vi "Get or Add Borders.vi"(8 "error in":errorcluster, 11 "SpreadsheetDoc in":refnum<k24>) -> (0 "error out":errorcluster, 2 "Borders":refnum<k24>, 3 "SpreadsheetDoc out":refnum<k24>)   [LabVIEW 2019, in "Open Xml.lvlib"]
uses:
  Open Xml.lvlib
  D:/git/Open-Xml-LabVIEW/Source/DocumentFormat.OpenXml.dll
  DocumentFormat.OpenXml.dll
  D:/git/Open-Xml-LabVIEW/Source/DocumentFormat.OpenXml.Framework.dll
  DocumentFormat.OpenXml.Framework.dll
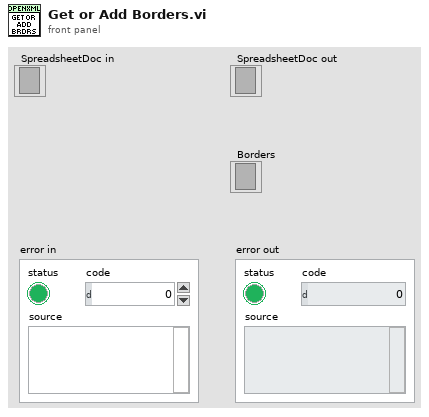
[diagram p1: front panel]
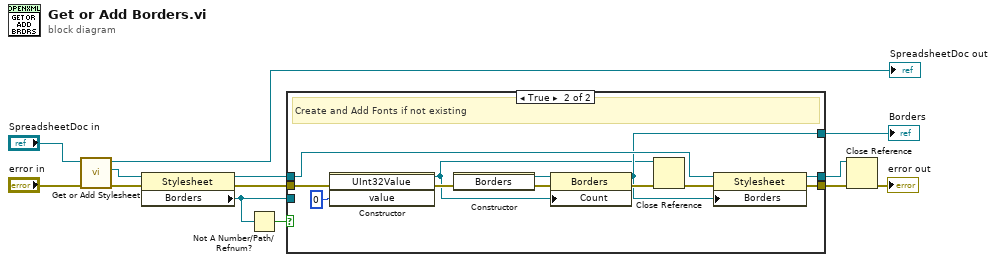
[diagram p0: block diagram]
diagram:
  n1 = call "Get or Add Stylesheet.vi"("error in"="error in", "SpreadsheetDoc in"="SpreadsheetDoc in") -> ("error out"=w12:errorcluster, "Stylesheet"=w9:refnum<k24>, "SpreadsheetDoc out"=→"SpreadsheetDoc out":refnum<k24>)  [unwired: 7 in]
  n2 = property class="Stylesheet"(reference=w9, error in=w12) -> (reference out=w7:refnum<k24>, error out=w10:errorcluster, "Borders"=w4:refnum<k24>)
  n3 = Not A Number/Path/Refnum?(number/path/refnum=w4) -> (NaN/Path/Refnum?=w8:bool)
  n4 = case shown="True" w8 {
    tunnel: w10 -> [w15 w22]
    tunnel: w7 -> [w14 w27]
    tunnel: [w15 w18] -> w6
    tunnel: w4 -> [w16 _]
    tunnel: [w16 w24] -> w3
    tunnel: [w14 w17] -> w1
    frame False {
      # "Fonts existing"
    }
    frame True {
      # "Create and Add Fonts if not existing"
      n5 = constructor class="UInt32Value"(error in=w22, "value"=u32 0) -> (reference out=w19:refnum<k24>, error out=w21:errorcluster)  [unwired: 2 in, 2 out]
      n6 = constructor class="Borders"(error in=w21) -> (reference out=w25:refnum<k24>, error out=w28:errorcluster)  [unwired: 2 in, 1 out]
      n7 = property class="Borders"(reference=w25, error in=w28, "Count"=w19) -> (reference out=w24:refnum<k24>, error out=w26:errorcluster)
      n8 = Close Reference(reference=w19, error in (no error)=w26) -> (error out=w20:errorcluster)
      n9 = property class="Stylesheet"(reference=w27, error in=w20, "Borders"=w24) -> (reference out=w17:refnum<k24>, error out=w18:errorcluster)
    }
  }
  "Borders" <- w3
  n10 = Close Reference(reference=w1, error in (no error)=w6) -> (error out=→"error out":errorcluster)
